vi "Deconstruct.vi"(0 "Build Analyzer":refnum<class "Build Analyzer.lvclass">, 11 "error in (no error)":errorcluster) -> (15 "error out":errorcluster)   [LabVIEW 2017, in "CL_G3_VIComponentBuilder.lvlib" / "Build Analyzer.lvclass"]
doc: "Destroys the working set."
uses:
  Build Analyzer.lvclass
  Build Analyzer.lvclass/Build Analyzer.ctl
  Accessors/Read Bubble Up Working Set.vi
  Accessors/Read Top Down Working Set.vi
  <userlib>/_Cirrus Logic/LabVIEW Container/Source/Container/Container.lvclass
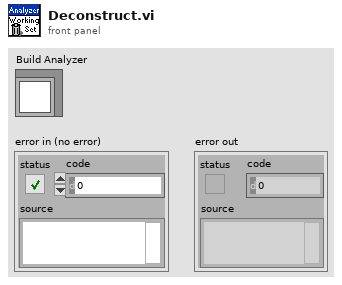
[diagram p1: front panel]
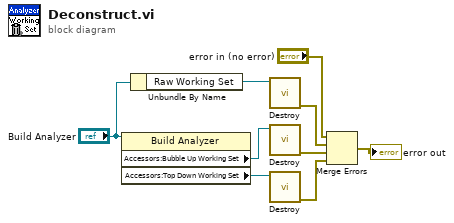
[diagram p0: block diagram]
diagram:
  n1 = property class="Build Analyzer"(reference="Build Analyzer") -> ("Accessors:Bubble Up Working Set"=w4:refnum<data-value>, "Accessors:Top Down Working Set"=w3:refnum<data-value>)  [unwired: 1 in, 2 out]
  n2 = Unbundle By Name("Build Analyzer") -> ("Raw Working Set"=w9:refnum<data-value>)
  n3 = call <userlib>:"Destroy.vi"("Container"=w9) -> ("error out"=w1:errorcluster)  [unwired: 10 in]
  n4 = call <userlib>:"Destroy.vi"("Container"=w4) -> ("error out"=w8:errorcluster)  [unwired: 10 in]
  n5 = call <userlib>:"Destroy.vi"("Container"=w3) -> ("error out"=w7:errorcluster)  [unwired: 10 in]
  n6 = Merge Errors("error in (no error)", w1, w8, w7) -> (→"error out":errorcluster)
